vi "Station Config to Tree Items.vi"(11 "Station Config":T2) -> (3 "Tree Items":T1(array[cluster]))   [LabVIEW 2025, in "Full User Interface.lvlib"]
uses:
  Full User Interface.lvlib
  Station Config.ctl
  Station Info.ctl
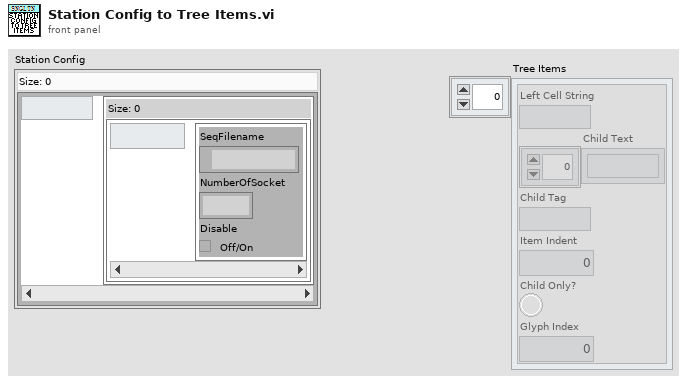
[diagram p1: front panel]
types:
  T1 = cluster{"Left Cell String":string, "Child Text":string[], "Child Tag":string, "Item Indent":i32, "Child Only?":bool, "Glyph Index":i32}[]
  T2 = typedef "Full User Interface.lvlib/Station Config.ctl" = map{string, map{i32, T3}}
  T3 = typedef "Full User Interface.lvlib/Station Info.ctl" = cluster{"SeqFilename":path, "NumberOfSocket":i32, "Disable":bool}
  T4 = cluster{"Left Cell String":string, "Child Text":string[], "Child Tag":string, "Item Indent":i32, "Child Only?":bool, "Glyph Index":i32}
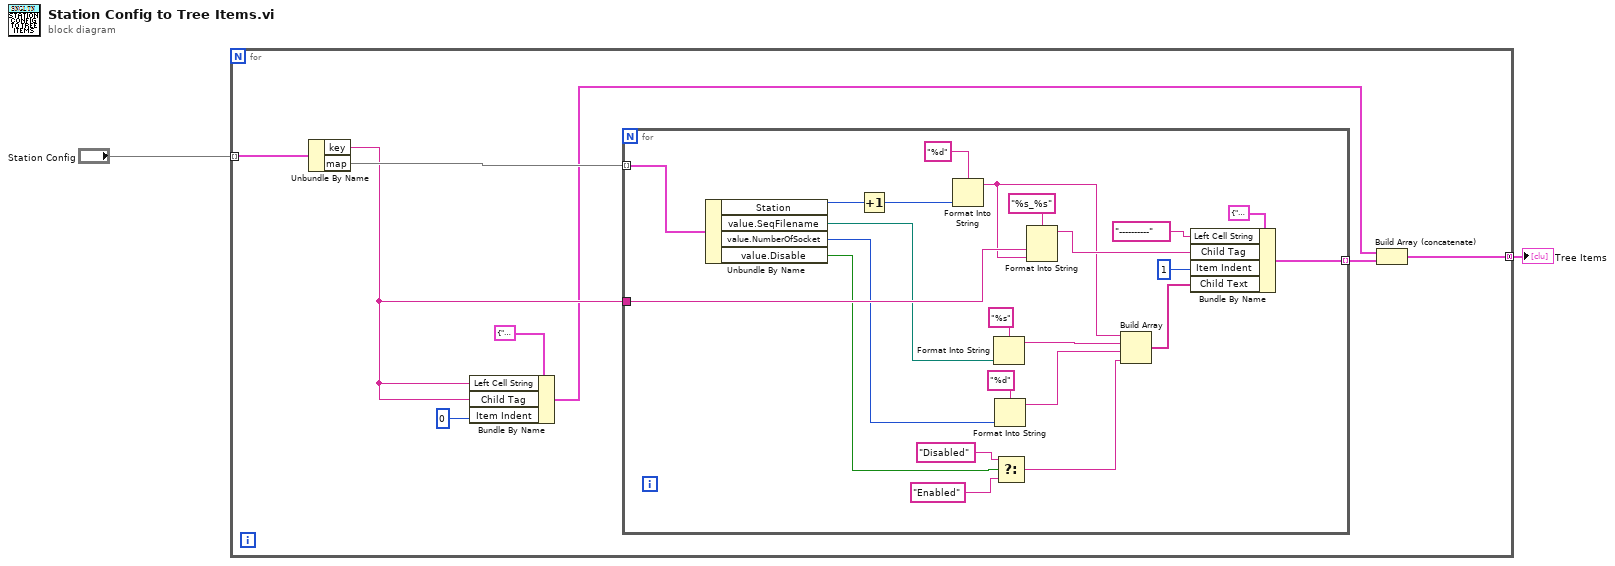
[diagram p0: block diagram]
diagram:
  n1 = for {
    tunnel: "Station Config" -> [w10] mode=indexing
    tunnel: [w3] -> w1 mode=concatenating
    n2 = Unbundle By Name(w10) -> ("key"=w6:string, "map"=w9:map{i32, T3})
    n3 = Bundle By Name(cluster=T4 {"Left Cell String"="", "Child Text"=[], "Child Tag"="", "Item Indent"=0, "Child Only?"=FALSE, "Glyph Index"=0} ("Item"), "Left Cell String"=w6, "Child Tag"=w6, "Item Indent"=0) -> (w4:T4)
    n4 = for {
      tunnel: w9 -> [w33] mode=indexing
      tunnel: w6 -> [w29]
      tunnel: [w18] -> w5 mode=indexing
      n5 = Unbundle By Name(w33) -> ("Station"=w31:i32, "value.SeqFilename"=w25:path, "value.NumberOfSocket"=w22:i32, "value.Disable"=w14:bool)
      n6 = Increment(x=w31) -> (x+1=w15:i32)
      n7 = Format Into String(format string="%d", w15) -> (resulting string=w17:string)  [unwired: 2 in, 1 out]
      n8 = Format Into String(format string="%s", w25) -> (resulting string=w21:string)  [unwired: 2 in, 1 out]
      n9 = Format Into String(format string="%d", w22) -> (resulting string=w20:string)  [unwired: 2 in, 1 out]
      n10 = Select(t="Disabled", s=w14, f="Enabled") -> (s? t:f=w11:string)
      n11 = Format Into String(format string="%s_%s", w29, w17) -> (resulting string=w27:string)  [unwired: 2 in, 1 out]
      n12 = Build Array(w17, w21, w20, w11) -> (w19:string[])
      n13 = Bundle By Name(cluster=T4 {"Left Cell String"="", "Child Text"=[], "Child Tag"="", "Item Indent"=0, "Child Only?"=FALSE, "Glyph Index"=0} ("Item"), "Left Cell String"="----------", "Child Tag"=w27, "Item Indent"=1, "Child Text"=w19) -> (w18:T4)
    }
    n14 = Build Array (concatenate)(w4, w5) -> (w3:T1)
  }
  "Tree Items" <- w1
